vi "_interfacebrowser Build MainTree Menu.vi"(7 "CtlRef":refnum<vi>, 9 "Coords":T1, 11 "Menu in":refnum<k9>) -> (3 "Discard?":bool)   [LabVIEW 2017]
uses:
  <vilib>/Utility/miscctls.llb/LVPoint32TypeDef.ctl
panel:
  out "Name(\"\" to use uuid) 2":string[](array[string])
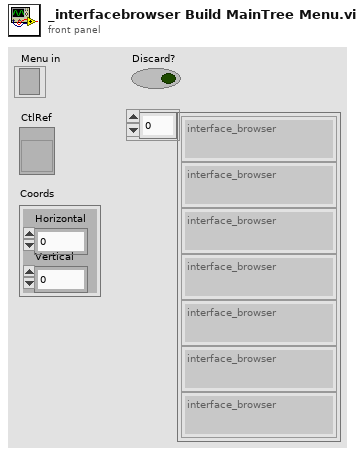
[diagram p1: front panel]
types:
  T1 = typedef "LVPoint32TypeDef.ctl" = cluster{"Horizontal":i32, "Vertical":i32}
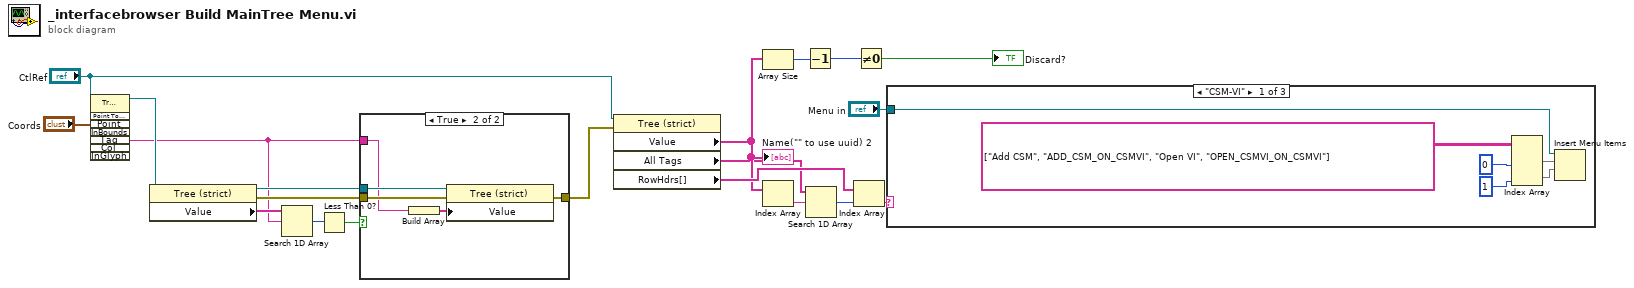
[diagram p0: block diagram]
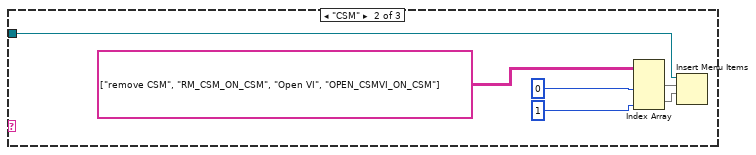
[diagram p3: hidden frame]
diagram:
  n1 = invoke on="Invoke Node" class="Tree (strict)" method="Point To Row Column"(reference="CtlRef", "Point"="Coords") -> (reference out=w8:refnum<vi>, "Tag"=w2:string)  [unwired: 6 in, 6 out]
  n2 = property on="Property Node" class="Tree (strict)"(reference=w8) -> (reference out=w4:refnum<vi>, error out=w5:errorcluster, "Value"=w7:string[])  [unwired: 1 in]
  n3 = Search 1D Array(1D array=w7, element=w2) -> (index of element=w6:i32)  [unwired: 1 in]
  n4 = Less Than 0?(x=w6) -> (x < 0?=w3:bool)
  n5 = case shown="True" w3 {
    tunnel: w5 -> [w21 w26]
    tunnel: w4 -> [_ w25]
    tunnel: w2 -> [_ w24]
    tunnel: [w21 w22] -> w1
    frame False {
    }
    frame True {
      n6 = Build Array(w24) -> (w23:string[])
      n7 = property on="Property Node" class="Tree (strict)"(reference=w25, error in=w26, "Value"=w23) -> (error out=w22:errorcluster)  [unwired: 1 out]
    }
  }
  n8 = property on="Property Node" class="Tree (strict)"(reference="CtlRef", error in=w1) -> ("Value"=w13:string[], "All Tags"=w12:string[], "RowHdrs[]"=w16:string[])  [unwired: 2 out]
  "Name(\"\" to use uuid) 2" <- w13
  n9 = Array Size(array=w13) -> (size(s)=w9:i32)
  n10 = Index Array(array=w13) -> (element=w14:string)  [unwired: 1 in]
  n11 = Decrement(x=w9) -> (x-1=w11:i32)
  n12 = Search 1D Array(1D array=w12, element=w14) -> (index of element=w15:i32)  [unwired: 1 in]
  n13 = Index Array(array=w16, index=w15) -> (element=w18:string)
  n14 = Not Equal To 0?(x=w11) -> (x != 0?=→"Discard?":bool)
  n15 = case shown="\"CSM-VI\"" w18 {
    tunnel: "Menu in" -> [w32 w38 _]
    frame "CSM-VI" {
      n16 = Index Array(array=string[][] [["Add CSM", "ADD_CSM_ON_CSMVI"], ["Open VI", "OPEN_CSMVI_ON_CSMVI"]] ("item names"), index (col) #1=0 ("disabled index (col)"), index (col) #2=1 ("index (col)")) -> (element #1=w30:string[], element #2=w29:string[])  [unwired: 2 in]
      n17 = Insert Menu Items(7:w29, 8:w30, 9:w32) -> ()  [unwired: 3 in, 3 out]
    }
    frame "CSM" {
      n18 = Index Array(array=string[][] [["remove CSM", "RM_CSM_ON_CSM"], ["Open VI", "OPEN_CSMVI_ON_CSM"]] ("item names"), index (col) #1=0 ("disabled index (col)"), index (col) #2=1 ("index (col)")) -> (element #1=w36:string[], element #2=w35:string[])  [unwired: 2 in]
      n19 = Insert Menu Items(7:w35, 8:w36, 9:w38) -> ()  [unwired: 3 in, 3 out]
    }
    frame "", Default {
    }
  }
